vi "AutoDrive.vi"(1 "Speed":dbl=1.0 format="%#_13g", 2 "Distance (ft)":dbl=10.0 format="%#_13g", 3 "Direction":T1(ring)) -> (0 "Distance (ft)":dbl(knob) scale=0.0..10.0)   [LabVIEW 2014]
panel:
  in  "Turn":dbl format="%#_13g"
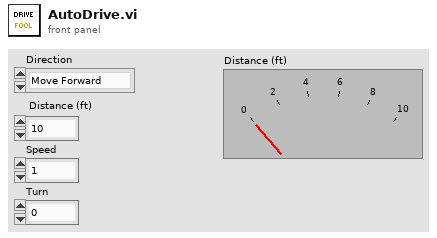
[diagram p1: front panel]
types:
  T1 = enum16{"Move Forward", "Move Backward", "Strafe Right", "Strafe Left"}
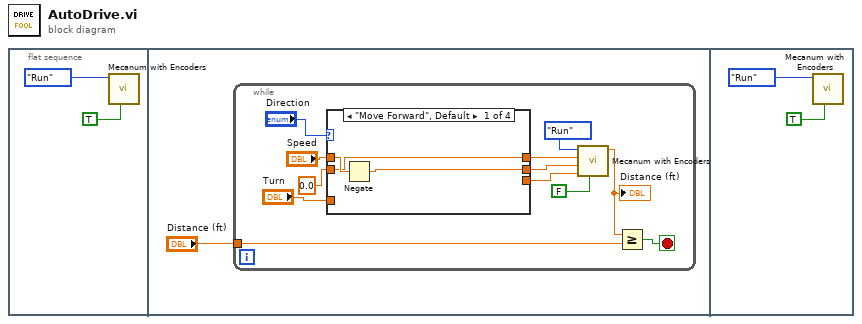
[diagram p0: block diagram]
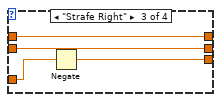
[diagram p3: hidden frame]
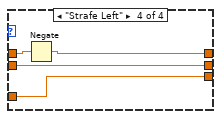
[diagram p4: hidden frame]
diagram:
  n1 = flat-sequence {
    frame #0 {
      n2 = call "Mecanum with Encoders.vi"("Reset"=TRUE, "Mode"=enum8{"Start", "Run", "Finish"}."Run") -> ()  [unwired: 8 in, 1 out]
    }
    frame #1 {
      n3 = while {
        tunnel: "Distance (ft)" -> [w8]
        stop <- w7 stop-if-true
        n4 = case shown="\"Move Forward\", Default" "Direction" {
          tunnel: [w16 w19 w23 w28] -> w13
          tunnel: "Speed" -> [w18 w19 w24 w27]
          tunnel: [w17 w20 w24 w26] -> w11
          tunnel: 0.0 ("Strafe") -> [w17 w20 w23 w28]
          tunnel: [_ _ w21 w25] -> w5
          tunnel: "Turn" -> [_ _ w22 w25]
          frame "Move Forward", Default {
            n5 = Negate(x=w18) -> (-x=w16:dbl)
          }
          frame "Move Backward" {
          }
          frame "Strafe Right" {
            n6 = Negate(x=w22) -> (-x=w21:dbl)
          }
          frame "Strafe Left" {
            n7 = Negate(x=w27) -> (-x=w26:dbl)
          }
        }
        n8 = call "Mecanum with Encoders.vi"("Reset"=FALSE, "Turn"=w5, "Forward/Backward"=w13, "Strafe"=w11, "Mode"=enum8{"Start", "Run", "Finish"}."Run") -> ("Distance (ft)"=w9:dbl)  [unwired: 5 in]
        "Distance (ft)" <- w9
        n9 = Greater Or Equal?(x=w9, y=w8) -> (x >= y?=w7:bool)
      }
    }
    frame #2 {
      n10 = call "Mecanum with Encoders.vi"("Reset"=TRUE, "Mode"=enum8{"Start", "Run", "Finish"}."Run") -> ()  [unwired: 8 in, 1 out]
    }
  }
